vi "footstep_metrics.vi"(6 "Start Index":i32, 9 "End Index":i32, 11 "Sensor Signal":dbl[][][](array[numeric])) -> (2 "Max Response":dbl[][](array[numeric]), 3 "Avg Response":dbl[][](array[numeric]))   [LabVIEW 2018]
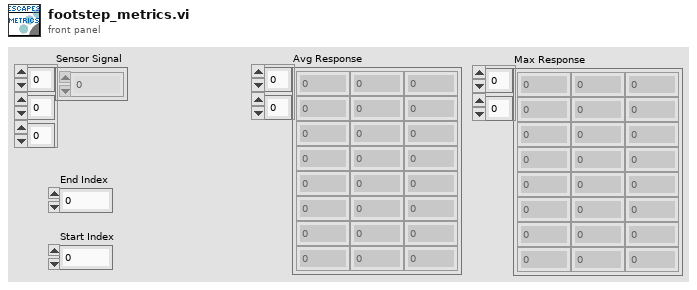
[diagram p1: front panel]
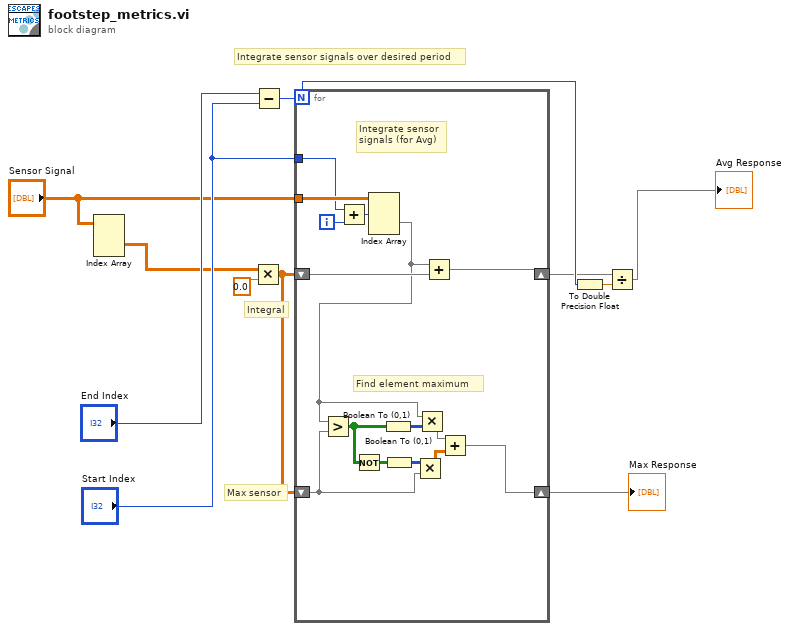
[diagram p0: block diagram]
diagram:
  # "Integral"
  # "Max sensor"
  # "Integrate sensor signals over desired period"
  n1 = Index Array(array="Sensor Signal") -> (element=w5:dbl[][])  [unwired: 3 in]
  n2 = Multiply(x=w5, y=0.0 ("Playback dT")) -> (x*y=w2:dbl[][])
  n3 = Subtract(x="End Index", y="Start Index") -> (x-y=w10:i32)
  n4 = for {
    N: w10 -> [_]
    tunnel: "Sensor Signal" -> [w26]
    tunnel: "Start Index" -> [w23]
    shift-right: [w22] -> w4
    shift-left: w2 -> [w21]
    shift-right: [w12] -> w1
    shift-left: w2 -> [w18]
    i -> [w25]
    # "Find element maximum"
    # "Integrate sensor\nsignals (for Avg)"
    n5 = Add(x=w23, y=w25) -> (x+y=w24:i32)
    n6 = Index Array(array=w26, index (dim 0)=w24) -> (element=w15:dbl[][])  [unwired: 2 in]
    n7 = Greater?(x=w15, y=w18) -> (0:w20:bool[][])
    n8 = Not(x=w20) -> (.not. x?=w19:bool[][])
    n9 = Boolean To (0,1)(Boolean=w20) -> (0, 1=w16:i16[][])
    n10 = Boolean To (0,1)(Boolean=w19) -> (0, 1=w17:i16[][])
    n11 = Multiply(x=w17, y=w18) -> (x*y=w13:dbl[][])
    n12 = Multiply(x=w15, y=w16) -> (x*y=w14:dbl[][])
    n13 = Add(x=w15, y=w21) -> (x+y=w22:dbl[][])
    n14 = Add(x=w14, y=w13) -> (x+y=w12:dbl[][])
  }
  "Max Response" <- w1
  n15 = To Double Precision Float(number=w10) -> (double precision float=w11:dbl)
  n16 = Divide(x=w4, y=w11) -> (x/y=→"Avg Response":dbl[][])
